vi "log_message.vi"(6 "timestamp":timestamp, 7 "context":string, 8 "error in (no error)":errorcluster, 9 "level":T1=400 items=["OFF"=0, "FATAL"=100, "ERROR"=200, "WARN"=300, "INFO"=400, "DEBUG"=500, "TRACE"=600, "ALL"=65535], 10 "message":string, 11 "File Log Provider in":refnum<class "File Log Provider.lvclass">) -> (0 "error out":errorcluster, 3 "File Log Provider out":refnum<class "File Log Provider.lvclass">)   [LabVIEW 2019, in "File Log Provider.lvclass"]
uses:
  File Log Provider.lvclass
  Queue Log Provider/Queue Log Provider.lvclass
  Log Service/public/level.ctl
  Log Service/Log Service.lvclass
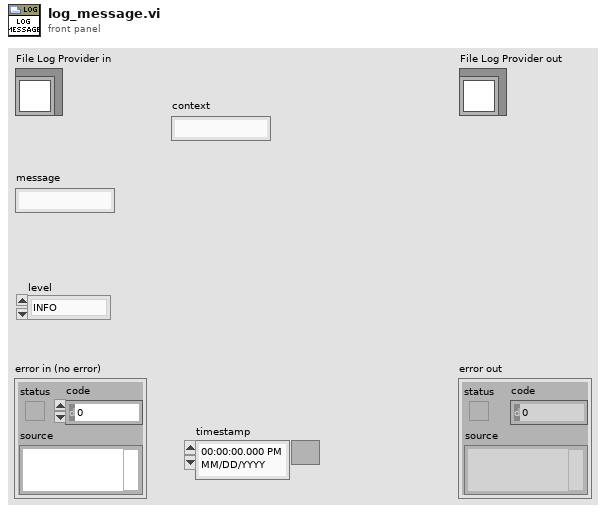
[diagram p1: front panel]
types:
  T1 = typedef "Utility API.lvlib/Log Service.lvclass/level.ctl" = u16
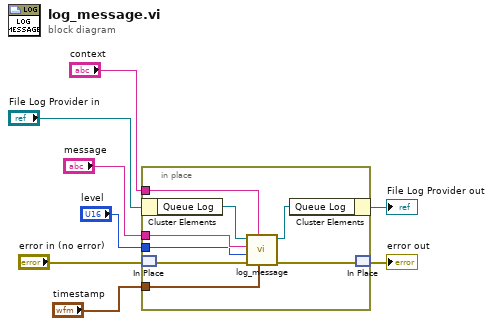
[diagram p0: block diagram]
diagram:
  n1 = in-place {
    in-place-border: "context" -> [w14]
    in-place-border: "message" -> [w13]
    in-place-border: "level" -> [w12]
    in-place-border: "timestamp" -> [w9]
    n2 = in-place-cluster #1("File Log Provider in") -> ("Queue Log"=w16:refnum<class "Queue Log Provider.lvclass">)
    n3 = in-place-match #2("error in (no error)") -> (w10:errorcluster)
    n4 = call-dynamic "log_message.vi"("timestamp"=w9, "context"=w14, "error in (no error)"=w10, "level"=w12, "message"=w13, "Queue Log Provider in"=w16) -> ("error out"=w11:errorcluster, "Queue Log Provider out"=w15:refnum<class "Queue Log Provider.lvclass">)  [unwired: 4 in]
    n5 = in-place-cluster #1("Queue Log"=w15) -> (→"File Log Provider out":refnum<class "File Log Provider.lvclass">)
    n6 = in-place-match #2(w11) -> (→"error out":errorcluster)
  }
